vi "WM_CAP - AM Capture.vi"() -> ()   [LabVIEW 2022 SP3]
uses:
  System.Windows.Forms
  user32.dll
  avicap32.dll
panel:
  in  "Preview":bool
  in  "Export":bool
  in  "Capture":bool
  in  "Frame to BMP":bool
  in  "Copy Frame":bool
  in  "Capture FPS":dbl
  in  "Preview FPS":dbl
  in  "PictureBox":refnum<k24>(container)
  out "Info":string
  in  "Fit Window":bool
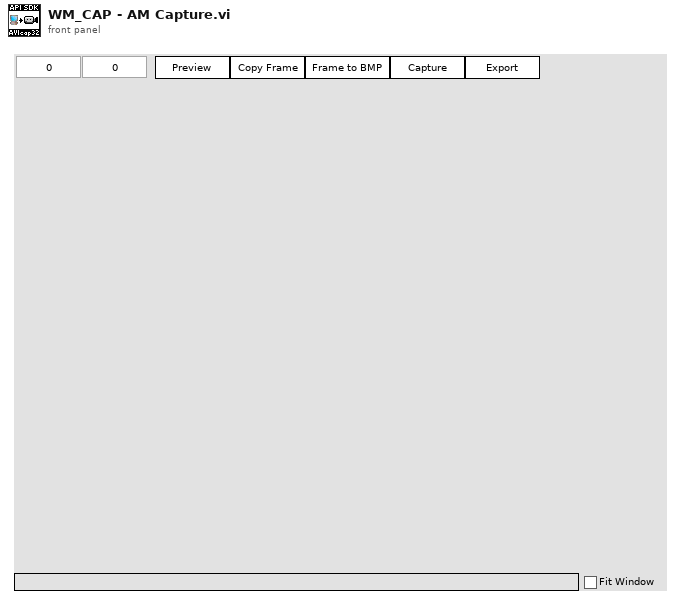
[diagram p1: front panel]
types:
  T1 = cluster{"biSize":i32, "biWidth":i32, "biHeight":i32, "biPlanes":i16, "biBitCount":i16, "biCompression":i32, "biSizeImage":i32, "biXPelsPerMeter":i32, "biYPelsPerMeter":i32, "biClrUsed":i32, "biClrImportant":i32, "Colors":u32[]}
  T2 = cluster{"uiImageWidth":u32, "uiImageHeight":u32, "fLiveWindow":u32, "fOverlayWindow":u32, "fScale":u32, "ptScroll":cluster{"x":i32, "y":i32}, "fUsingDefaultPalette":u32, "fAudioHardware":u32, "fCapFileExists":u32, "dwCurrentVideoFrame":u32, "dwCurrentVideoFramesDropped":u32, "dwCurrentWaveSamples":u32, "dwCurrentTimeElapsedMS":u32, "hPalCurrent":u32, "fCapturingNow":u32, "dwReturn":u32, "wNumVideoAllocated":u32, "wNumAudioAllocated":u32}
  T3 = cluster{"Timeout":i32, "Error":errorcluster, "hwnd":u32, "WM_CAP_START":u32, "CAPSTATUS":cluster{"uiImageWidth":u32, "uiImageHeight":u32, "fLiveWindow":u32, "fOverlayWindow":u32, "fScale":u32, "ptScroll":cluster{"x":i32, "y":i32}, "fUsingDefaultPalette":u32, "fAudioHardware":u32, "fCapFileExists":u32, "dwCurrentVideoFrame":u32, "dwCurrentVideoFramesDropped":u32, "dwCurrentWaveSamples":u32, "dwCurrentTimeElapsedMS":u32, "hPalCurrent":u32, "fCapturingNow":u32, "dwReturn":u32, "wNumVideoAllocated":u32, "wNumAudioAllocated":u32}, "BITMAPINFO":cluster{"biSize":i32, "biWidth":i32, "biHeight":i32, "biPlanes":i16, "biBitCount":i16, "biCompression":i32, "biSizeImage":i32, "biXPelsPerMeter":i32, "biYPelsPerMeter":i32, "biClrUsed":i32, "biClrImportant":i32, "Colors":u32[]}, "Preview FPS":dbl, "Capture FPS":dbl, "Camera":string}
  T4 = typedef "sizeaction.ctl" = enum32{"Minimized", "Maximized", "Resized"}
  T5 = typedef "LVRectTypeDef.ctl" = cluster{"Left":i16, "Top":i16, "Right":i16, "Bottom":i16}
  T6 = cluster{"wDeviceIndex":u32, "fHasOverlay":u32, "fHasDlgVideoSource":u32, "fHasDlgVideoFormat":u32, "fHasDlgVideoDisplay":u32, "fCaptureInitialized":u32, "fDriverSuppliesPalettes":u32, "hVideoIn":u32, "hVideoOut":u32, "hVideoExtIn":u32, "hVideoExtOut":u32}
  T7 = typedef "imagedata.ctl" = cluster{"image type":i32, "image depth":i32, "image":u8[], "mask":u8[], "colors":u32[], "Rectangle":cluster{"left":i16, "top":i16, "right":i16, "bottom":i16}}
  T8 = cluster{"dwRequestMicroSecPerFrame":u32, "fMakeUserHitOKToCapture":u32, "wPercentDropForError":u32, "fYield":u32, "dwIndexSize":u32, "wChunkGranularity":u32, "fUsingDOSMemory":u32, "wNumVideoRequested":u32, "fCaptureAudio":u32, "wNumAudioRequested":u32, "vKeyAbort":u32, "fAbortLeftMouse":u32, "fAbortRightMouse":u32, "fLimitEnabled":u32, "wTimeLimit":u32, "fMCIControl":u32, "fStepMCIDevice":u32, "dwMCIStartTime":u32, "dwMCIStopTime":u32, " fStepCaptureAt2x":u32, "wStepCaptureAverageFrames":u32, "dwAudioBufferSize":u32, "fDisableWriteCache":u32, "AVStreamMaster":u32}
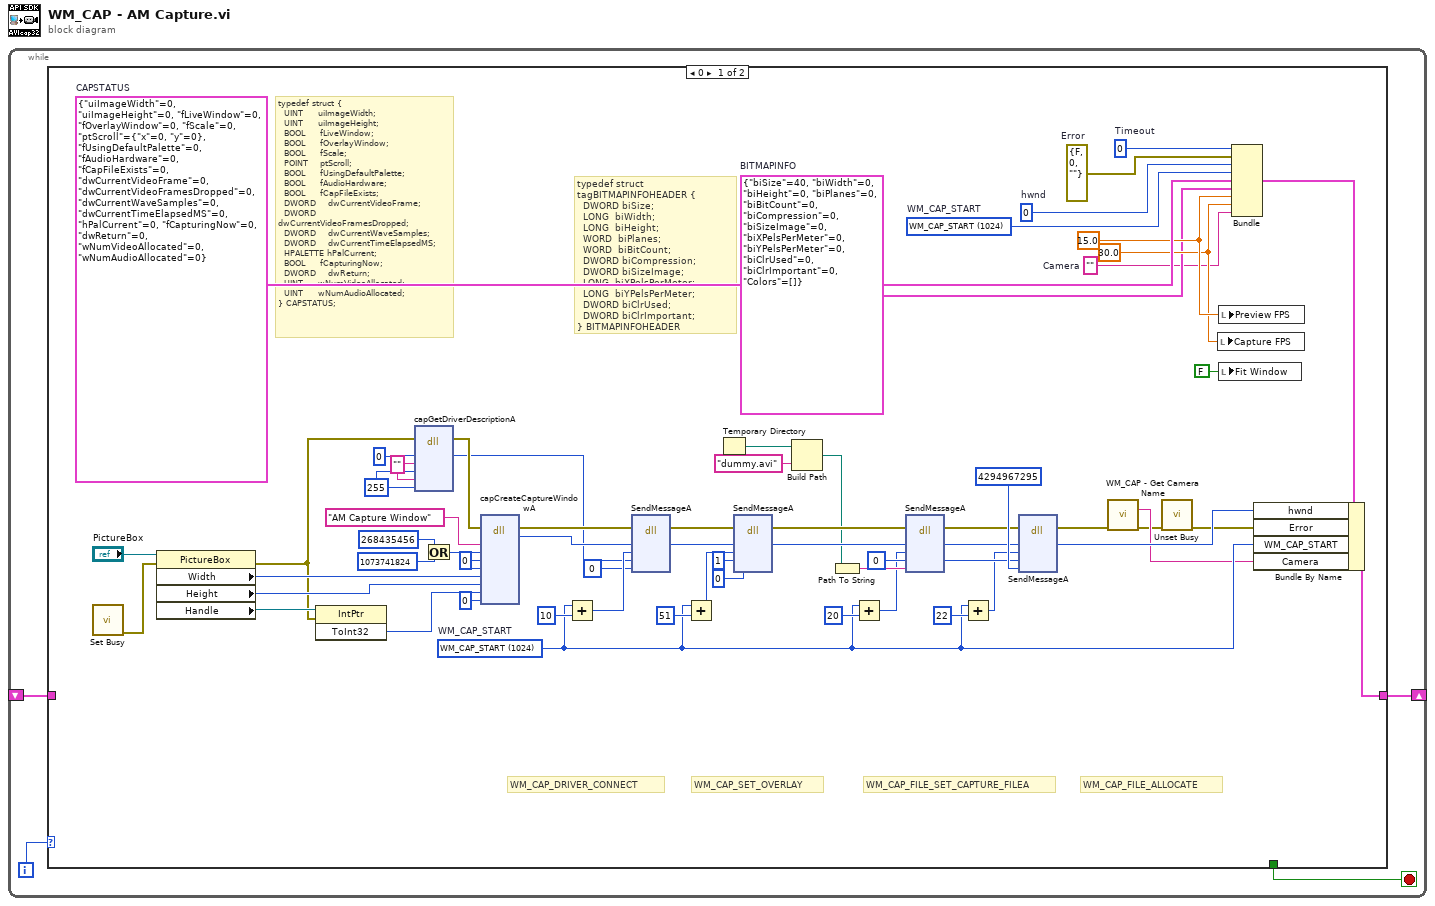
[diagram p0: block diagram]
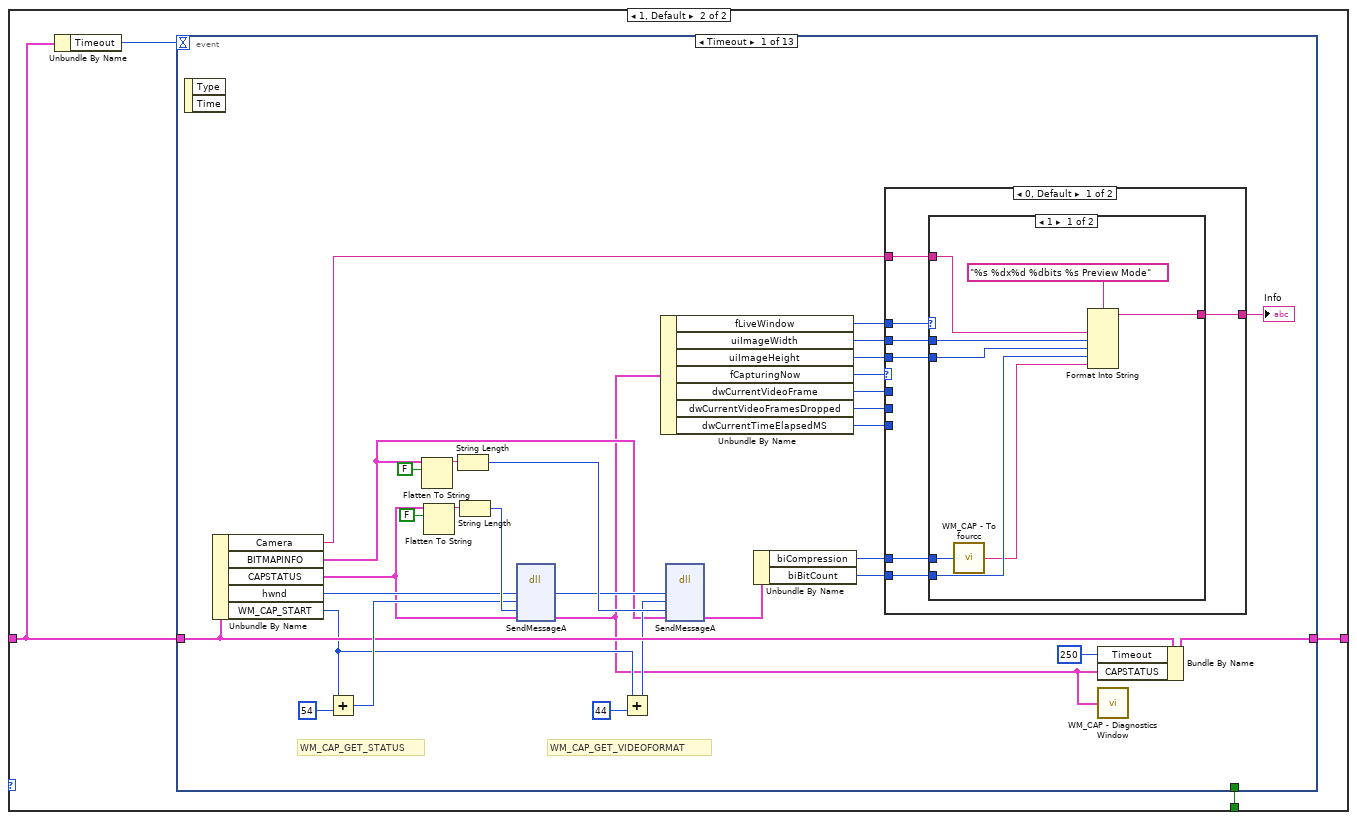
[diagram p2: hidden frame]
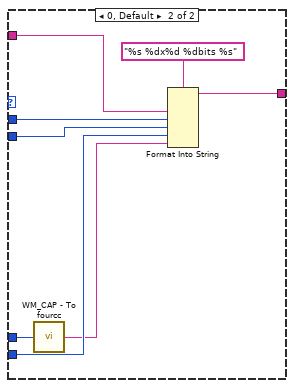
[diagram p3: hidden frame]
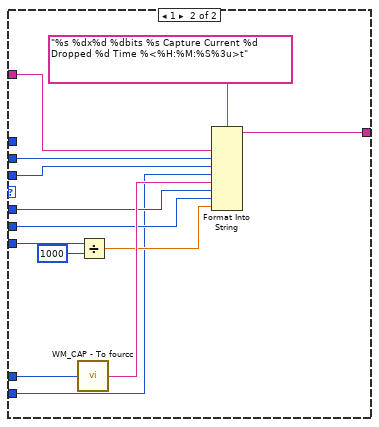
[diagram p4: hidden frame]
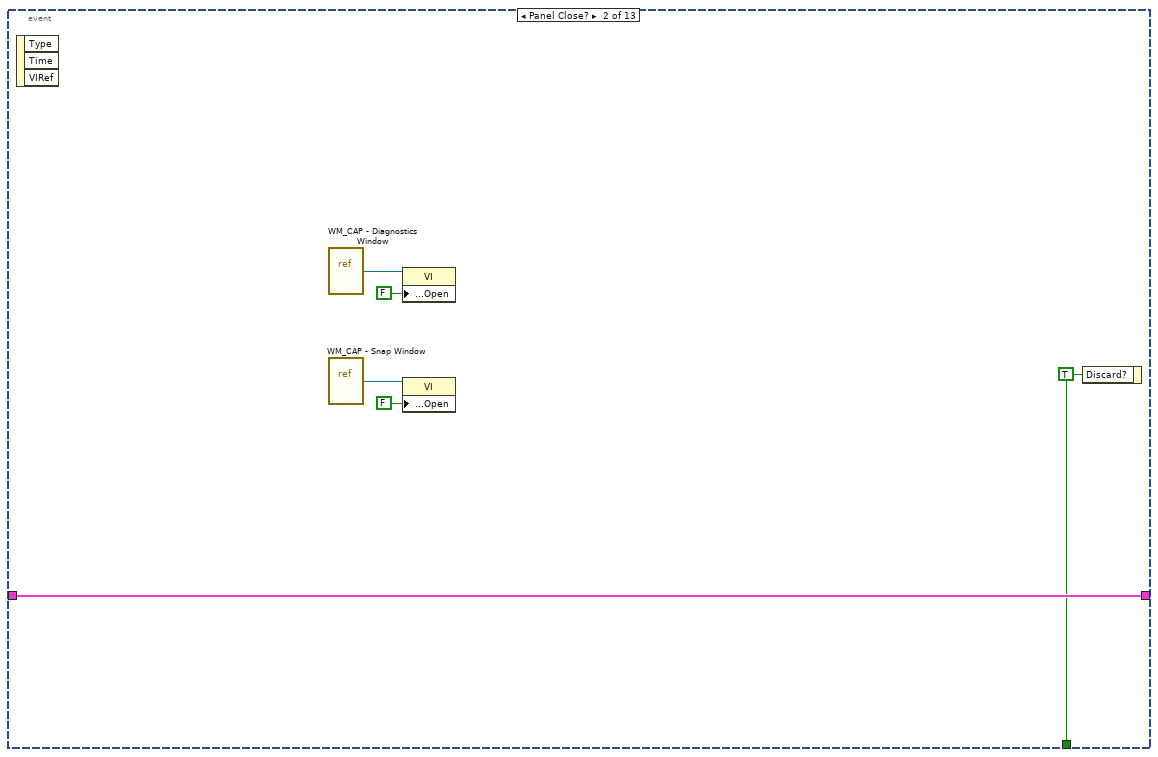
[diagram p5: hidden frame]
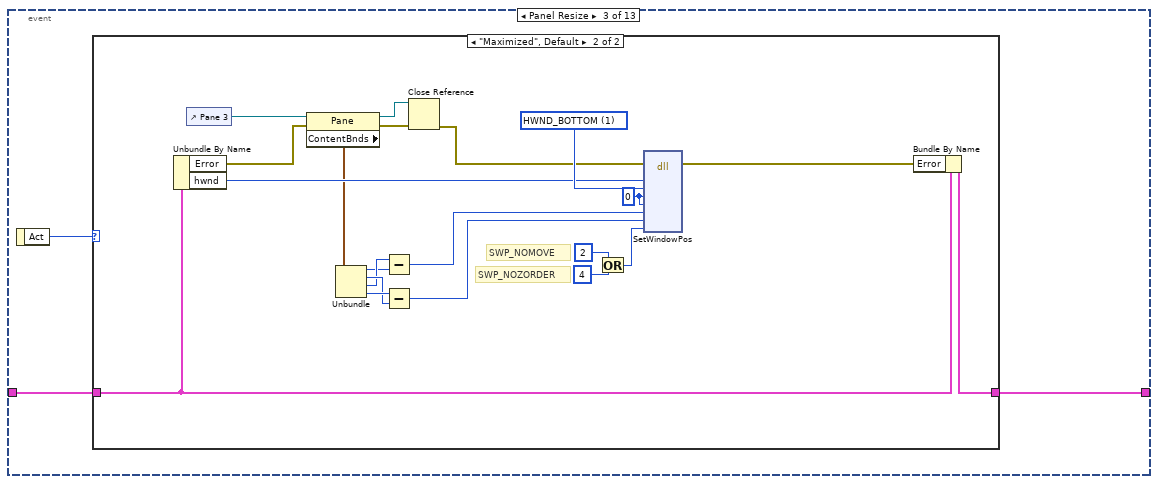
[diagram p6: hidden frame]
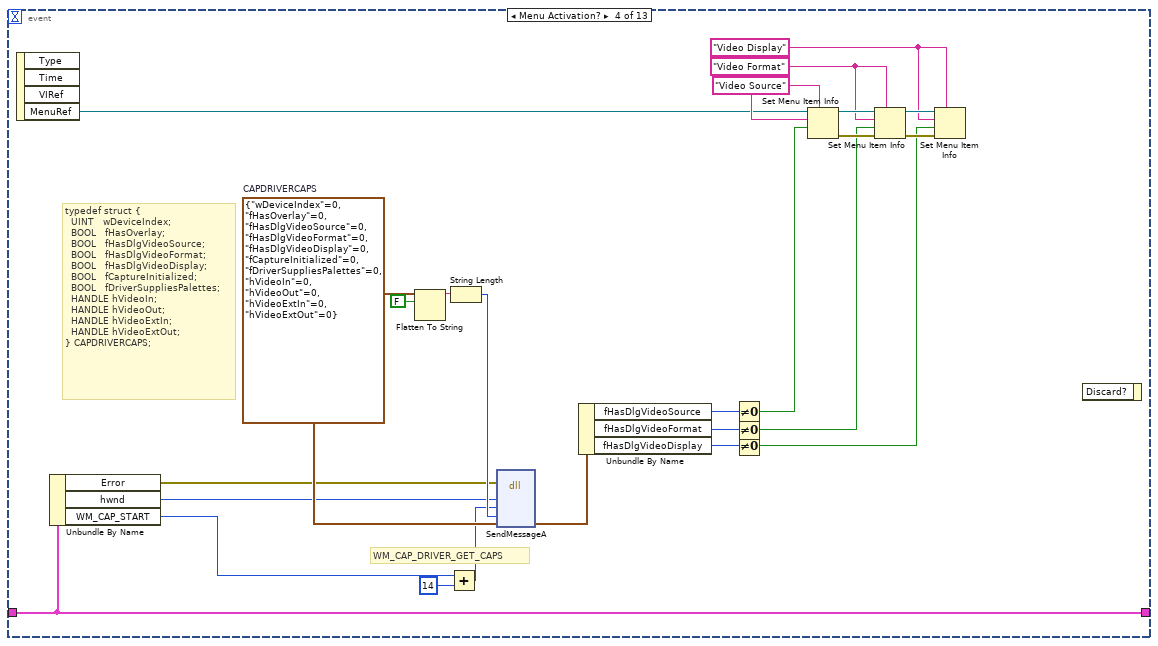
[diagram p8: hidden frame]
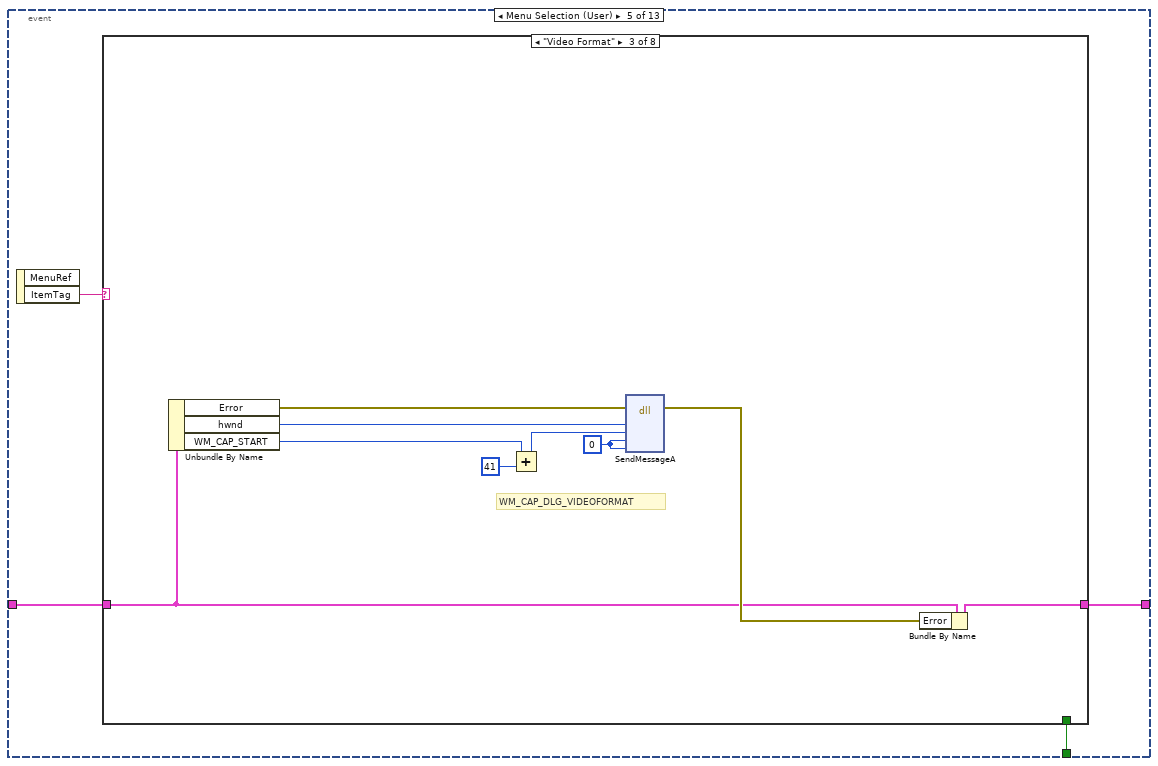
[diagram p9: hidden frame]
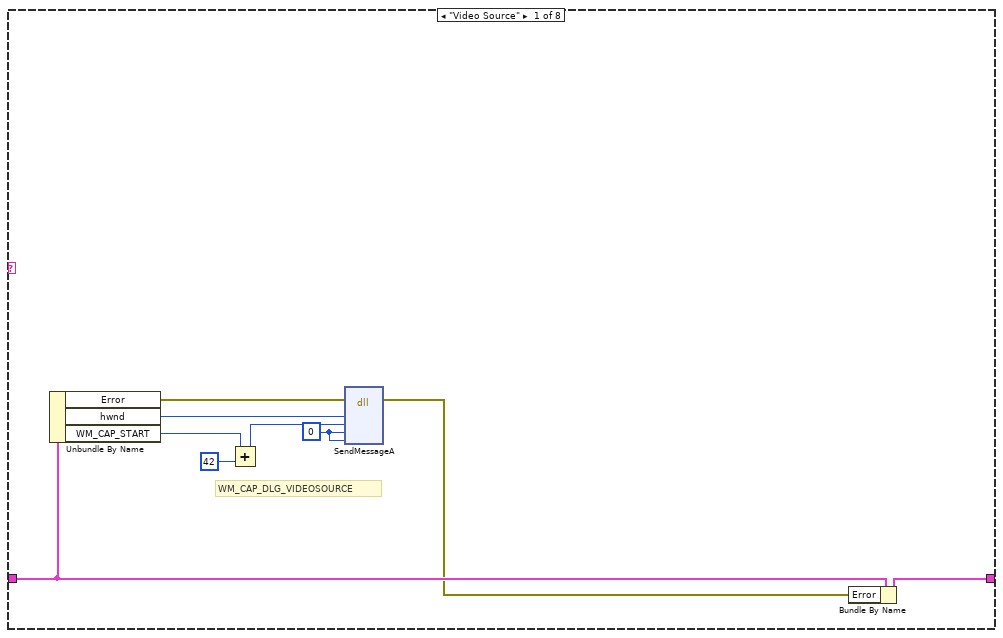
[diagram p10: hidden frame]
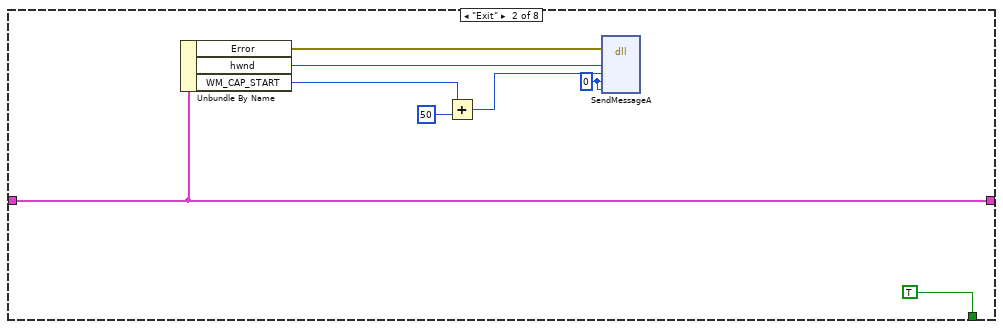
[diagram p11: hidden frame]
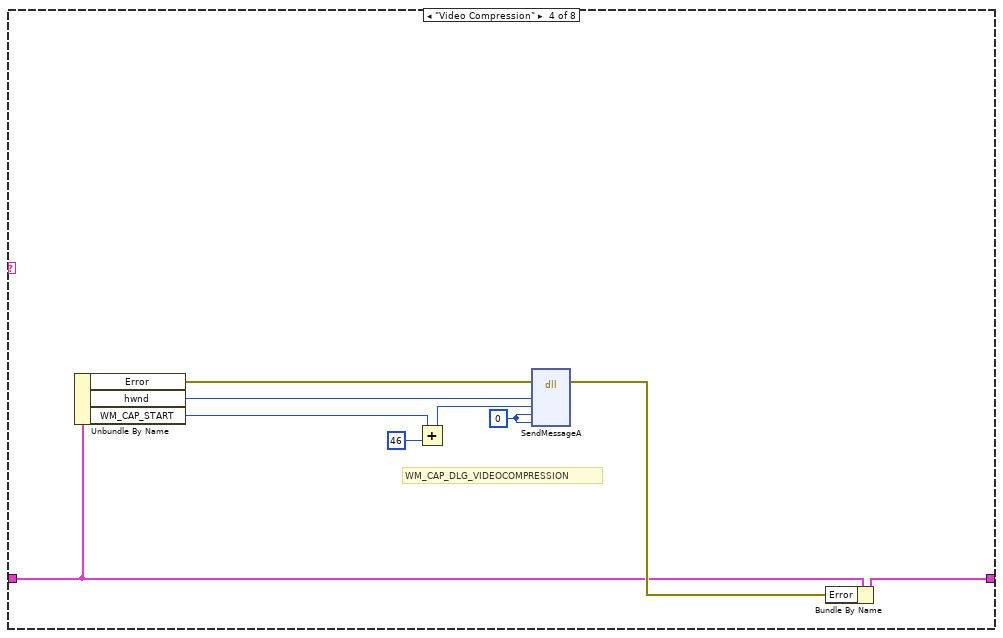
[diagram p12: hidden frame]
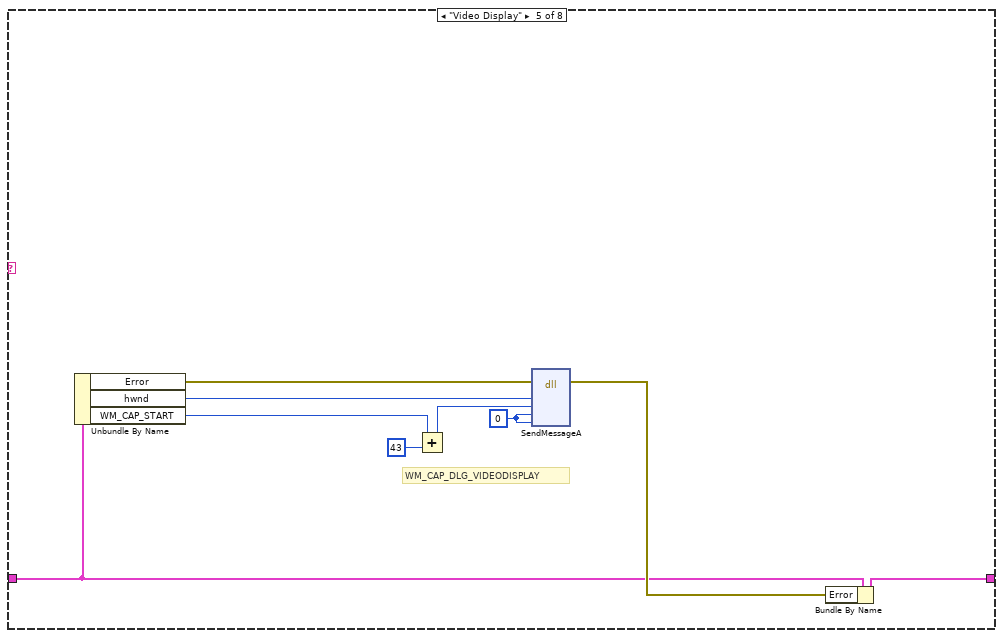
[diagram p13: hidden frame]
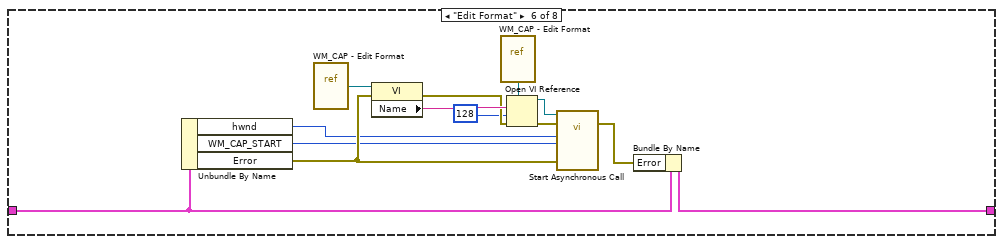
[diagram p14: hidden frame]
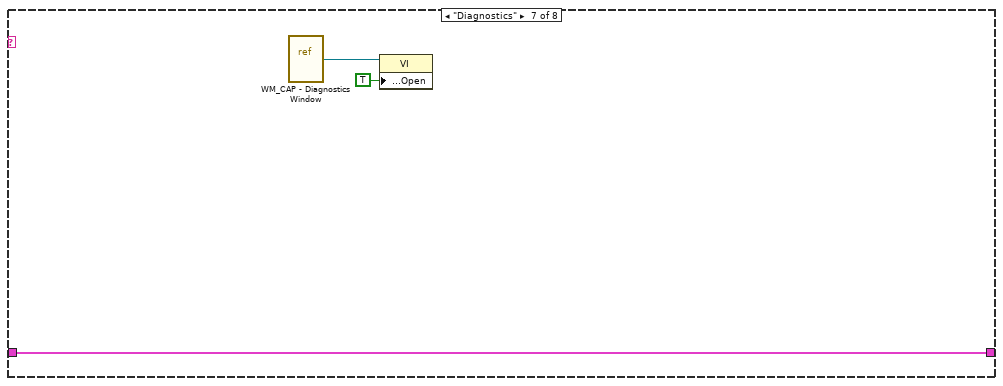
[diagram p15: hidden frame]
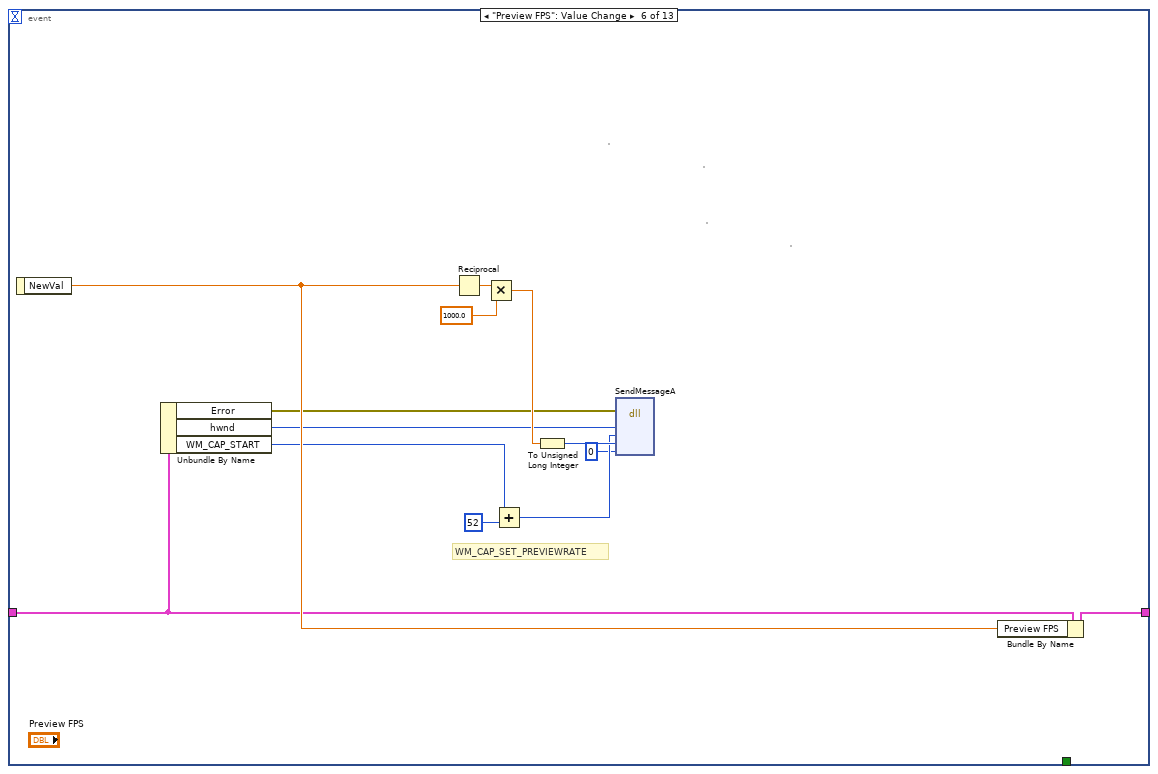
[diagram p17: hidden frame]
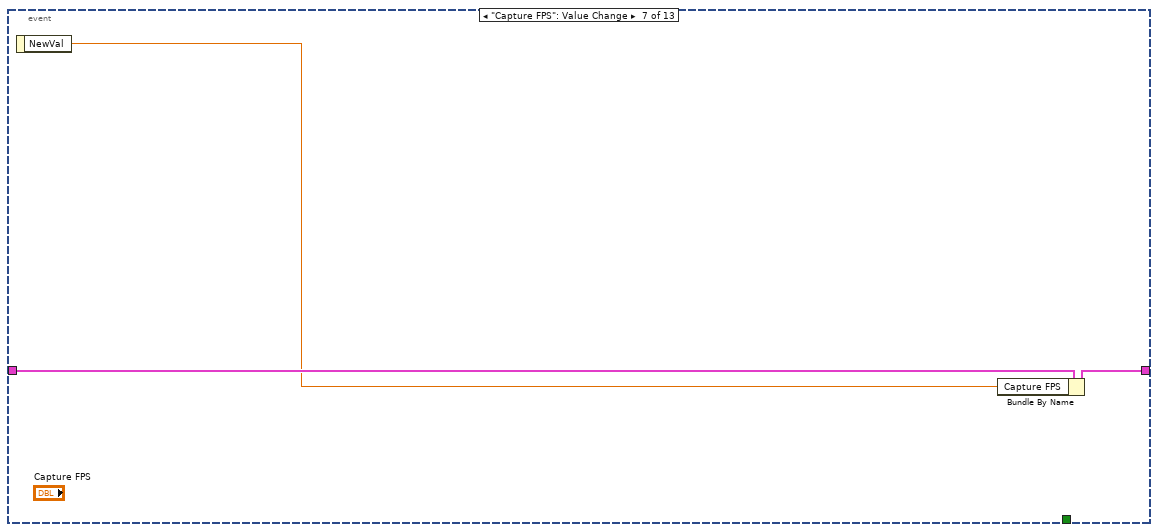
[diagram p18: hidden frame]
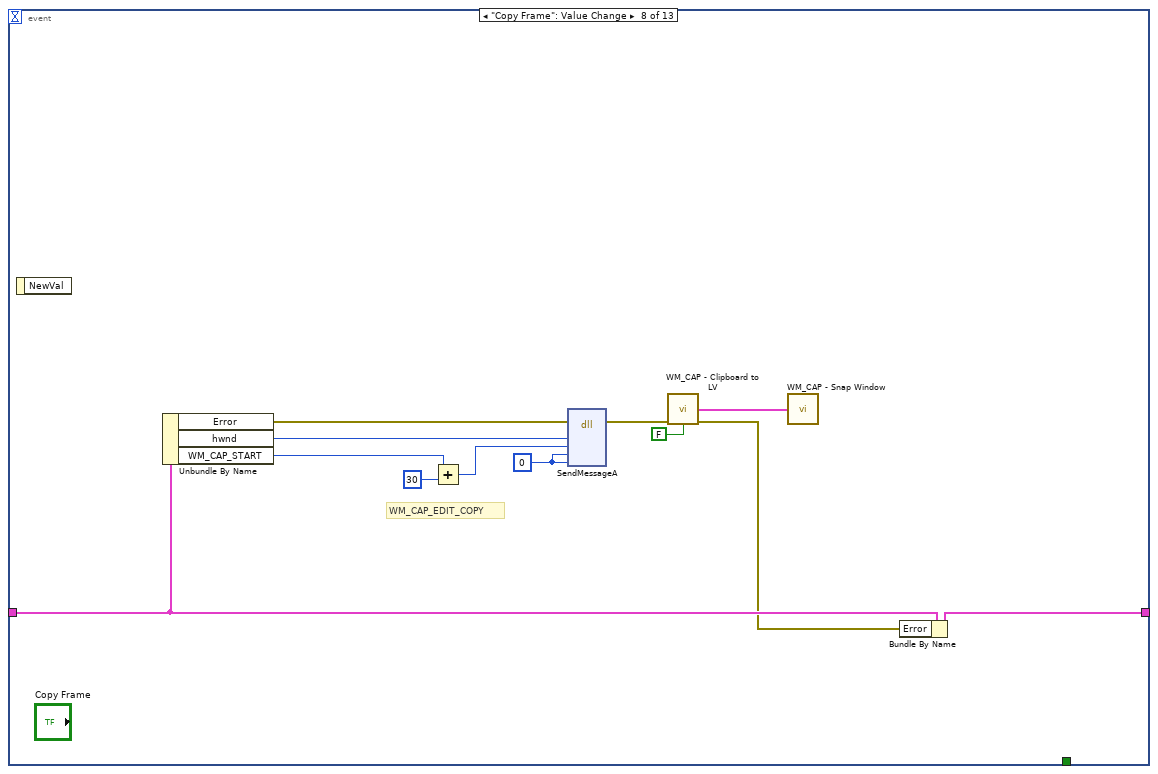
[diagram p19: hidden frame]
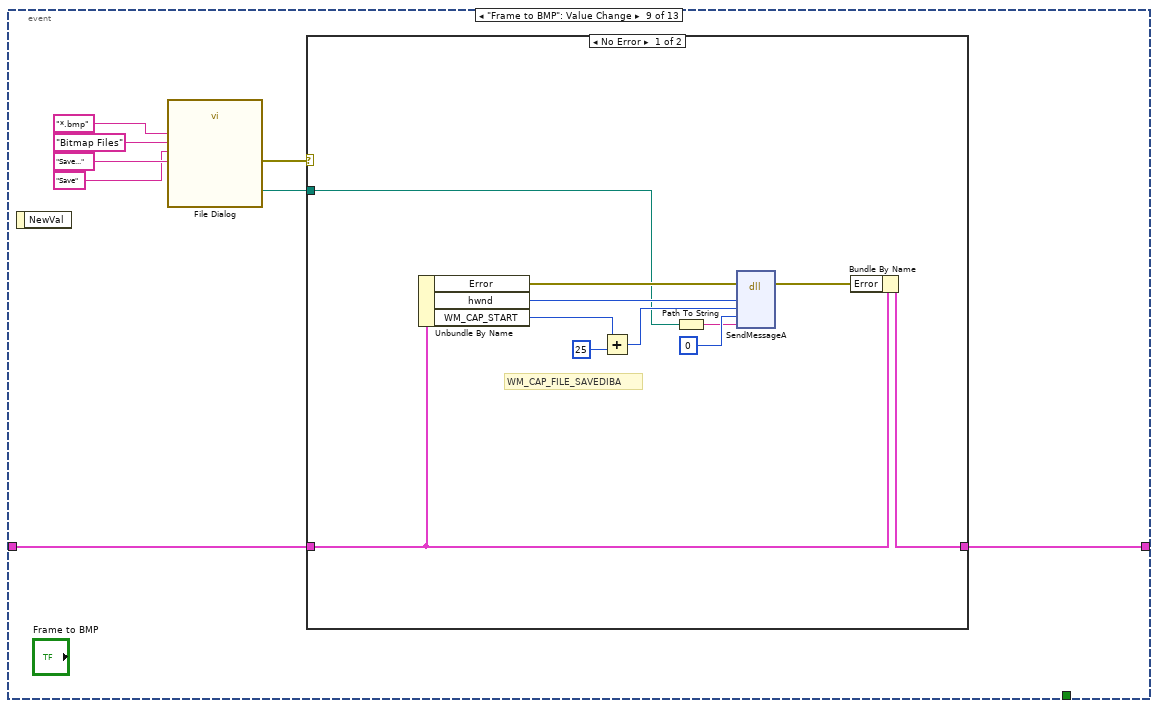
[diagram p20: hidden frame]
diagram:
  n1 = while {
    shift-right: [w3] -> _
    shift-left: _ -> [w2]
    i -> [w4]
    stop <- w1 stop-if-true
    n2 = case shown="0" w4 {
      tunnel: [w47 w70] -> w3
      tunnel: w2 -> [_ w69]
      tunnel: [_ w67] -> w1
      frame 0 {
        w8 = ""  # Camera
        w12 = T1 {"biSize"=40, "biWidth"=0, "biHeight"=0, "biPlanes"=0, "biBitCount"=0, "biCompression"=0, "biSizeImage"=0, "biXPelsPerMeter"=0, "biYPelsPerMeter"=0, "biClrUsed"=0, "biClrImportant"=0, "Colors"=[]}  # BITMAPINFO
        w17 = T2 {"uiImageWidth"=0, "uiImageHeight"=0, "fLiveWindow"=0, "fOverlayWindow"=0, "fScale"=0, "ptScroll"={"x"=0, "y"=0}, "fUsingDefaultPalette"=0, "fAudioHardware"=0, "fCapFileExists"=0, "dwCurrentVideoFrame"=0, "dwCurrentVideoFramesDropped"=0, "dwCurrentWaveSamples"=0, "dwCurrentTimeElapsedMS"=0, "hPalCurrent"=0, "fCapturingNow"=0, "dwReturn"=0, "wNumVideoAllocated"=0, "wNumAudioAllocated"=0}  # CAPSTATUS
        w14 = 30.0 ("Capture FPS")
        w15 = 15.0 ("Preview FPS")
        w22 = u32 1024 items=["WM_CAP_START"=1024]  # WM_CAP_START
        w23 = u32 1024 items=["WM_CAP_START"=1024]  # WM_CAP_START
        w48 = u32 0  # hwnd
        w55 = u32 0 ("x")
        w61 = 255 ("cbName")
        w62 = ""
        w65 = errorcluster {"status"=FALSE, "code"=0, "source"=""}  # Error
        w66 = 0  # Timeout
        # "typedef struct tagBITMAPINFOHEADER {\n  DWORD biSize;\n  LONG  biWidth;\n  LONG  biHeight;\n  WORD  biPlanes;\n  WORD  biBitCount;\n  DWORD biCompression;\n  DWORD biSizeImage;\n  LONG  biXPelsPerMeter;\n  LONG  biYPelsPerMeter;\n  DWORD biClrUsed;\n  DWORD biClrImportant;\n} BITMAPINFOHEADER"
        # "typedef struct {\n  UINT     uiImageWidth;\n  UINT     uiImageHeight;\n  BOOL     fLiveWindow;\n  BOOL     fOverlayWindow;\n  BOOL     fScale;\n  POINT    ptScroll;\n  BOOL     fUsingDefaultPalette;\n  BOOL     fAudioHardware;\n  BOOL     fCapFileExists;\n  DWORD    dwCurrentVideoFrame;\n  DWORD    dwCurrentVideoFramesDropped;\n  DWORD    dwCurrentWaveSamples;\n  DWORD    dwCurrentTimeElapsedMS;\n  HPALETTE hPalCurrent;\n  BOOL     fCapturingNow;\n  DWORD    dwReturn;\n  UINT     wNumVideoAllocated;\n  UINT     wNumAudioAllocated;\n} CAPSTATUS;"
        # "WM_CAP_FILE_ALLOCATE"
        # "WM_CAP_FILE_SET_CAPTURE_FILEA"
        # "WM_CAP_SET_OVERLAY"
        # "WM_CAP_DRIVER_CONNECT"
        n3 = call <vilib>:"Set Busy.vi"() -> ("error out"=w19:errorcluster)  [unwired: 10 in, 1 out]
        n4 = property class="PictureBox"(reference="PictureBox", error in=w19) -> (error out=w16:errorcluster, "Width"=w59:i32, "Height"=w60:i32, "Handle"=w57:refnum<k24>)  [unwired: 1 out]
        n5 = invoke class="IntPtr" method="ToInt32"(reference=w57, error in=w16) -> ("ToInt32"=w58:i32)  [unwired: 1 in, 2 out]
        n6 = dll-call lib="avicap32.dll" fn="capGetDriverDescriptionA"(error in=w16, "wDriverIndex"=0, "lpszName"=w62, "cbName"=w61, "lpszVer"=w62, "cbVer"=w61) -> (error out=w49:errorcluster, "wDriverIndex"=w20:i32)  [unwired: 7 in, 1 out]
        n7 = Or(x=u32 268435456, y=u32 1073741824) -> (x .or. y?=w54:u32)
        n8 = dll-call lib="avicap32.dll" fn="capCreateCaptureWindowA"(error in=w49, "lpszWindowName"="AM Capture Window", "dwStyle"=w54, "x"=w55, "y"=w55, "nWidth"=w59, "nHeight"=w60, "hwnd"=w58, "nID"=u32 0) -> (error out=w46:errorcluster, "return type"=w44:u32)  [unwired: 10 in, 1 out]
        n9 = Add(x=w23, y=u32 10) -> (x+y=w43:u32)
        n10 = dll-call lib="user32.dll" fn="SendMessageA"(error in=w46, "hwnd"=w44, "msg"=w43, "wParam"=w20, "lparam"=u32 0 ("msg")) -> (error out=w39:errorcluster, "hwnd"=w37:u32)  [unwired: 6 in, 1 out]
        n11 = Add(x=w23, y=u32 51) -> (x+y=w36:u32)
        n12 = Temporary Directory() -> (w11:path)
        n13 = dll-call lib="user32.dll" fn="SendMessageA"(error in=w39, "hwnd"=w37, "msg"=w36, "wParam"=u32 1, "lparam"=u32 0) -> (error out=w25:errorcluster, "hwnd"=w21:u32)  [unwired: 6 in, 1 out]
        n14 = Build Path(base path=w11, name or relative path="dummy.avi") -> (appended path=w9:path)
        n15 = Path To String(path=w9) -> (string=w29:string)
        n16 = Add(x=w23, y=u32 20) -> (x+y=w27:u32)
        n17 = dll-call lib="user32.dll" fn="SendMessageA"(error in=w25, "hwnd"=w21, "msg"=w27, "wParam"=u32 0 ("msg"), "lparam"=w29) -> (error out=w30:errorcluster, "hwnd"=w31:u32, "wParam"=w34:u32)  [unwired: 5 in, 1 out]
        n18 = Add(x=w23, y=u32 22) -> (x+y=w33:u32)
        n19 = dll-call lib="user32.dll" fn="SendMessageA"(error in=w30, "hwnd"=w31, "msg"=w33, "wParam"=w34, "lparam"=u32 4294967295) -> (error out=w6:errorcluster, "hwnd"=w24:u32)  [unwired: 6 in, 1 out]
        n20 = call "WM_CAP - Get Camera Name.vi"("error in (no error)"=w6) -> ("FriendlyName"=w7:string, "error out"=w5:errorcluster)  [unwired: 12 in, 1 out]
        n21 = call <vilib>:"Unset Busy.vi"("error in (no error)"=w5) -> ("error out"=w18:errorcluster)  [unwired: 10 in]
        n22 = local write "Capture FPS"(w14) -> ()
        n23 = local write "Preview FPS"(w15) -> ()
        n24 = local write "Fit Window"(FALSE ("Fit Window")) -> ()
        n25 = Bundle("Timeout"=w66, "Error"=w65, "hwnd"=w48, "WM_CAP_START"=w22, "CAPSTATUS"=w17, "BITMAPINFO"=w12, "Preview FPS"=w15, "Capture FPS"=w14, "Camera"=w8) -> (w64:T3)  [unwired: 1 in]
        n26 = Bundle By Name(cluster=w64, "hwnd"=w24, "Error"=w18, "WM_CAP_START"=w23, "Camera"=w7) -> (w47:T3)
      }
      frame 1, Default {
        n27 = Unbundle By Name(w69) -> ("Timeout"=w68:i32)
        n28 = event shown="[0] Timeout" {
          selector: _ -> [_ _ _ _ _ _ _ _ _ _ _ _ _]
          dyn-events: _ -> [_ _ _ _ _ _ _ _ _ _ _ _ _]
          timeout: w68 -> [_ _ _ _ _ _ _ _ _ _ _ _ _]
          tunnel: [w101 w143 w145 w184 w196 w271 w273 w279 w293 w308 w361 w381 w415] -> w70
          tunnel: w69 -> [w94 w143 w146 w184 w195 w262 w274 w283 w294 w309 w362 w382 w415]
          tunnel: [_ w142 _ _ w194 _ _ _ _ _ _ _ _] -> w67
          event Timeout {
            # "WM_CAP_GET_VIDEOFORMAT"
            # "WM_CAP_GET_STATUS"
            n29 = event-data() -> ()  [unwired: 1 in, 2 out]
            n30 = Unbundle By Name(w94) -> ("Camera"=w71:string, "BITMAPINFO"=w81:T1, "CAPSTATUS"=w92:T2, "hwnd"=w93:u32, "WM_CAP_START"=w82:u32)
            n31 = Add(x=w82, y=u32 54) -> (x+y=w96:u32)
            n32 = Flatten To String(anything=w81, prepend array or string size? (T)=FALSE) -> (data string=w87:string)  [unwired: 2 in, 2 out]
            n33 = Flatten To String(anything=w92, prepend array or string size? (T)=FALSE) -> (data string=w97:string)  [unwired: 2 in, 2 out]
            n34 = String Length(string=w87) -> (length=w85:i32)
            n35 = String Length(string=w97) -> (length=w99:i32)
            n36 = dll-call lib="user32.dll" fn="SendMessageA"("hwnd"=w93, "msg"=w96, "wParam"=w99, w92) -> ("hwnd"=w83:u32, w80:T2)  [unwired: 6 in, 2 out]
            n37 = Add(x=w82, y=u16 44) -> (x+y=w84:u32)
            n38 = Unbundle By Name(w80) -> ("fLiveWindow"=w75:u32, "uiImageWidth"=w90:u32, "uiImageHeight"=w89:u32, "fCapturingNow"=w91:u32, "dwCurrentVideoFrame"=w74:u32, "dwCurrentVideoFramesDropped"=w73:u32, "dwCurrentTimeElapsedMS"=w72:u32)
            n39 = dll-call lib="user32.dll" fn="SendMessageA"("hwnd"=w83, "msg"=w84, "wParam"=w85, "lparam"=w81) -> ("lparam"=w79:T1)  [unwired: 7 in, 2 out]
            n40 = Unbundle By Name(w79) -> ("biCompression"=w78:i32, "biBitCount"=w77:i16)
            n41 = case shown="0, Default" w91 {
              tunnel: w90 -> [w108 w131]
              tunnel: w89 -> [w107 w130]
              tunnel: w78 -> [w105 w137]
              tunnel: w77 -> [w106 w125]
              tunnel: [w104 w136] -> w76
              tunnel: w75 -> [w103 _]
              tunnel: w74 -> [_ w126]
              tunnel: w73 -> [_ w127]
              tunnel: w72 -> [_ w134]
              tunnel: w71 -> [w102 w132]
              frame 0, Default {
                n42 = case shown="1" w103 {
                  tunnel: w108 -> [w112 w120]
                  tunnel: w107 -> [w111 w119]
                  tunnel: w106 -> [w110 w118]
                  tunnel: w105 -> [w115 w123]
                  tunnel: [w114 w122] -> w104
                  tunnel: w102 -> [w113 w121]
                  frame 1 {
                    n43 = call "WM_CAP - To fourcc.vi"("biCompression"=w115) -> ("FOURCC"=w109:string)  [unwired: 14 in]
                    n44 = Format Into String(format string="%s %dx%d %dbits %s Preview Mode", w113, w112, w111, w110, w109) -> (resulting string=w114:string)  [unwired: 2 in, 1 out]
                  }
                  frame 0, Default {
                    n45 = call "WM_CAP - To fourcc.vi"("biCompression"=w123) -> ("FOURCC"=w117:string)  [unwired: 14 in]
                    n46 = Format Into String(format string="%s %dx%d %dbits %s", w121, w120, w119, w118, w117) -> (resulting string=w122:string)  [unwired: 2 in, 1 out]
                  }
                }
              }
              frame 1 {
                n47 = call "WM_CAP - To fourcc.vi"("biCompression"=w137) -> ("FOURCC"=w129:string)  [unwired: 14 in]
                n48 = Divide(x=w134, y=u32 1000) -> (x/y=w128:dbl)
                n49 = Format Into String(format string="%s %dx%d %dbits %s Capture Current %d Dropped %d Time %<%H:%M:%S%3u>t", w132, w131, w130, w125, w129, w126, w127, w128) -> (resulting string=w136:string)  [unwired: 2 in, 1 out]
              }
            }
            "Info" <- w76
            n50 = Bundle By Name(cluster=w94, "Timeout"=250, "CAPSTATUS"=w80) -> (w101:T3)
            n51 = call "WM_CAP - Diagnostics Window.vi"("CAPSTATUS In"=w80) -> ()  [unwired: 15 in]
          }
          event Panel Close? {
            w142 = TRUE ("Discard?")
            n52 = event-data() -> ()  [unwired: 1 in, 3 out]
            n53 = vi-ref "WM_CAP - Diagnostics Window.vi"() -> (w141:refnum<vi>)
            n54 = vi-ref "WM_CAP - Snap Window.vi"() -> (w138:refnum<vi>)
            n55 = property class="VI"(reference=w141, "Front Panel.Open"=FALSE ("Front Panel Window:Open")) -> ()  [unwired: 1 in, 2 out]
            n56 = property class="VI"(reference=w138, "Front Panel.Open"=FALSE ("Front Panel Window:Open")) -> ()  [unwired: 1 in, 2 out]
            n57 = event-data("Discard?"=w142) -> ()  [unwired: 1 in, 1 out]
          }
          event Panel Resize {
            n58 = event-data() -> ("Act"=w144:T4)  [unwired: 1 in]
            n59 = case shown="\"Maximized\", Default" w144 {
              tunnel: w146 -> [w147 w164]
              tunnel: [w147 w162] -> w145
              frame "Minimized" {
              }
              frame "Maximized", Default {
                w151 = u32 0 ("x")
                w167 = 1 items=["HWND_BOTTOM"=1, "HWND_NOTOPMOST"=-2, "HWND_TOP"=0, "HWND_TOPMOST"=-1] ("hwndInsertAfter")
                # "SWP_NOMOVE"
                # "SWP_NOZORDER"
                n60 = Unbundle By Name(w164) -> ("Error"=w155:errorcluster, "hwnd"=w163:u32)
                n61 = control-ref of="Pane 3"() -> (w148:refnum<vi>)
                n62 = property class="Pane"(reference=w148, error in=w155) -> (reference out=w154:refnum<vi>, error out=w153:errorcluster, "ContentBnds"=w160:T5)
                n63 = Unbundle(w160) -> ("Left"=w156:i16, "Top"=w158:i16, "Right"=w157:i16, "Bottom"=w159:i16)
                n64 = Subtract(x=w157, y=w156) -> (x-y=w150:i16)
                n65 = Subtract(x=w159, y=w158) -> (x-y=w149:i16)
                n66 = Close Reference(reference=w154, error in (no error)=w153) -> (error out=w152:errorcluster)
                n67 = Or(x=u32 2, y=u32 4) -> (x .or. y?=w168:u32)
                n68 = dll-call lib="user32.dll" fn="SetWindowPos"(error in=w152, "hwnd"=w163, "hwndInsertAfter"=w167, "x"=w151, "y"=w151, "cx"=w150, "cy"=w149, "uFlags"=w168) -> (error out=w161:errorcluster)  [unwired: 10 in, 1 out]
                n69 = Bundle By Name(cluster=w164, "Error"=w161) -> (w162:T3)
              }
            }
          }
          event Menu Activation? {
            w176 = "Video Display" ("item tag")
            w177 = "Video Format" ("item tag")
            w178 = "Video Source" ("item tag")
            w192 = T6 {"wDeviceIndex"=0, "fHasOverlay"=0, "fHasDlgVideoSource"=0, "fHasDlgVideoFormat"=0, "fHasDlgVideoDisplay"=0, "fCaptureInitialized"=0, "fDriverSuppliesPalettes"=0, "hVideoIn"=0, "hVideoOut"=0, "hVideoExtIn"=0, "hVideoExtOut"=0}  # CAPDRIVERCAPS
            # "WM_CAP_DRIVER_GET_CAPS"
            # "typedef struct {\n  UINT   wDeviceIndex;\n  BOOL   fHasOverlay;\n  BOOL   fHasDlgVideoSource;\n  BOOL   fHasDlgVideoFormat;\n  BOOL   fHasDlgVideoDisplay;\n  BOOL   fCaptureInitialized;\n  BOOL   fDriverSuppliesPalettes;\n  HANDLE hVideoIn;\n  HANDLE hVideoOut;\n  HANDLE hVideoExtIn;\n  HANDLE hVideoExtOut;\n} CAPDRIVERCAPS;"
            n70 = event-data() -> ("MenuRef"=w169:refnum<k9>)  [unwired: 1 in, 3 out]
            n71 = Unbundle By Name(w184) -> ("Error"=w187:errorcluster, "hwnd"=w186:u32, "WM_CAP_START"=w185:u32)
            n72 = Flatten To String(anything=w192, prepend array or string size? (T)=FALSE) -> (data string=w190:string)  [unwired: 2 in, 2 out]
            n73 = Add(x=w185, y=u32 14) -> (x+y=w189:u32)
            n74 = String Length(string=w190) -> (length=w193:i32)
            n75 = dll-call lib="user32.dll" fn="SendMessageA"(error in=w187, "hwnd"=w186, "msg"=w189, "wParam"=w193, "lparam"=w192) -> ("lparam"=w181:T6)  [unwired: 6 in, 2 out]
            n76 = Unbundle By Name(w181) -> ("fHasDlgVideoSource"=w175:u32, "fHasDlgVideoFormat"=w174:u32, "fHasDlgVideoDisplay"=w173:u32)
            n77 = Not Equal To 0?(x=w175) -> (x != 0?=w172:bool)
            n78 = Not Equal To 0?(x=w174) -> (x != 0?=w171:bool)
            n79 = Not Equal To 0?(x=w173) -> (x != 0?=w170:bool)
            n80 = Set Menu Item Info(7:w178, 9:w172, 10:w178, 11:w169) -> (0:w183:errorcluster, 3:w180:refnum<k9>)  [unwired: 3 in]
            n81 = Set Menu Item Info(7:w177, 8:w183, 9:w171, 10:w177, 11:w180) -> (0:w182:errorcluster, 3:w179:refnum<k9>)  [unwired: 2 in]
            n82 = Set Menu Item Info(7:w176, 8:w182, 9:w170, 10:w176, 11:w179) -> ()  [unwired: 2 in, 2 out]
            n83 = event-data() -> ()  [unwired: 2 in, 1 out]
          }
          event Menu Selection (User) {
            n84 = event-data() -> ("ItemTag"=w197:string)  [unwired: 1 in, 1 out]
            n85 = case shown="\"Video Format\"" w197 {
              tunnel: [w201 w211 w220 w229 w238 w253 w257 w258] -> w196
              tunnel: w195 -> [w203 w211 w218 w227 w236 w254 w257 w258]
              tunnel: [_ TRUE _ _ _ _ _ _] -> w194
              frame "Video Source" {
                w206 = u32 0 ("msg")
                # "WM_CAP_DLG_VIDEOSOURCE"
                n86 = Unbundle By Name(w203) -> ("Error"=w199:errorcluster, "hwnd"=w198:u32, "WM_CAP_START"=w202:u32)
                n87 = Add(x=w202, y=u32 42) -> (x+y=w205:u32)
                n88 = dll-call lib="user32.dll" fn="SendMessageA"(error in=w199, "hwnd"=w198, "msg"=w205, "wParam"=w206, "lparam"=w206) -> (error out=w200:errorcluster)  [unwired: 7 in, 1 out]
                n89 = Bundle By Name(cluster=w203, "Error"=w200) -> (w201:T3)
              }
              frame "Exit" {
                w207 = u32 0 ("wParam")
                n90 = Unbundle By Name(w211) -> ("Error"=w210:errorcluster, "hwnd"=w209:u32, "WM_CAP_START"=w208:u32)
                n91 = Add(x=w208, y=u32 50) -> (x+y=w213:u32)
                n92 = dll-call lib="user32.dll" fn="SendMessageA"(error in=w210, "hwnd"=w209, "msg"=w213, "wParam"=w207, "lparam"=w207) -> ()  [unwired: 7 in, 2 out]
              }
              frame "Video Format" {
                w223 = u32 0 ("msg")
                # "WM_CAP_DLG_VIDEOFORMAT"
                n93 = Unbundle By Name(w218) -> ("Error"=w215:errorcluster, "hwnd"=w216:u32, "WM_CAP_START"=w217:u32)
                n94 = Add(x=w217, y=u32 41) -> (x+y=w222:u32)
                n95 = dll-call lib="user32.dll" fn="SendMessageA"(error in=w215, "hwnd"=w216, "msg"=w222, "wParam"=w223, "lparam"=w223) -> (error out=w219:errorcluster)  [unwired: 7 in, 1 out]
                n96 = Bundle By Name(cluster=w218, "Error"=w219) -> (w220:T3)
              }
              frame "Video Compression" {
                w232 = u32 0 ("msg")
                # "WM_CAP_DLG_VIDEOCOMPRESSION"
                n97 = Unbundle By Name(w227) -> ("Error"=w224:errorcluster, "hwnd"=w225:u32, "WM_CAP_START"=w226:u32)
                n98 = Add(x=w226, y=u32 46) -> (x+y=w231:u32)
                n99 = dll-call lib="user32.dll" fn="SendMessageA"(error in=w224, "hwnd"=w225, "msg"=w231, "wParam"=w232, "lparam"=w232) -> (error out=w228:errorcluster)  [unwired: 7 in, 1 out]
                n100 = Bundle By Name(cluster=w227, "Error"=w228) -> (w229:T3)
              }
              frame "Video Display" {
                w241 = u32 0 ("msg")
                # "WM_CAP_DLG_VIDEODISPLAY"
                n101 = Unbundle By Name(w236) -> ("Error"=w233:errorcluster, "hwnd"=w234:u32, "WM_CAP_START"=w235:u32)
                n102 = Add(x=w235, y=u32 43) -> (x+y=w240:u32)
                n103 = dll-call lib="user32.dll" fn="SendMessageA"(error in=w233, "hwnd"=w234, "msg"=w240, "wParam"=w241, "lparam"=w241) -> (error out=w237:errorcluster)  [unwired: 7 in, 1 out]
                n104 = Bundle By Name(cluster=w236, "Error"=w237) -> (w238:T3)
              }
              frame "Edit Format" {
                n105 = Unbundle By Name(w254) -> ("hwnd"=w243:u32, "WM_CAP_START"=w242:u32, "Error"=w244:errorcluster)
                n106 = vi-ref "WM_CAP - Edit Format.vi"() -> (w252:refnum<vi>)
                n107 = property class="VI"(reference=w252, error in=w244) -> (error out=w250:errorcluster, "Name"=w251:string)  [unwired: 1 out]
                n108 = vi-ref "WM_CAP - Edit Format.vi"() -> (w249:refnum<vi>)
                n109 = Open VI Reference(type specifier VI Refnum (for type only)=w249, vi path=w251, options=128, error in (no error)=w250) -> (vi reference=w246:refnum<vi>, error out=w247:errorcluster)  [unwired: 2 in]
                n110 = call-by-ref "Start Asynchronous Call"(reference=w246, error in=w247, "hwnd"=w243, "WM_CAP_START"=w242, "Error"=w244) -> (error out=w245:errorcluster)  [unwired: 12 in, 2 out]
                n111 = Bundle By Name(cluster=w254, "Error"=w245) -> (w253:T3)
              }
              frame "Diagnostics" {
                n112 = vi-ref "WM_CAP - Diagnostics Window.vi"() -> (w256:refnum<vi>)
                n113 = property class="VI"(reference=w256, "Front Panel.Open"=TRUE ("Front Panel Window:Open")) -> ()  [unwired: 1 in, 2 out]
              }
              frame "Error", Default {
              }
            }
          }
          event "Preview FPS": Value Change {
            # "WM_CAP_SET_PREVIEWRATE"
            n114 = event-data() -> ("NewVal"=w263:dbl)  [unwired: 1 in]
            n115 = Unbundle By Name(w262) -> ("Error"=w261:errorcluster, "hwnd"=w260:u32, "WM_CAP_START"=w259:u32)
            n116 = Reciprocal(x=w263) -> (1/x=w267:dbl)
            n117 = Multiply(x=w267, y=1000.0) -> (x*y=w269:dbl)
            n118 = Add(x=w259, y=u32 52) -> (x+y=w266:u32)
            n119 = To Unsigned Long Integer(number=w269) -> (unsigned 32bit integer=w270:u32)
            n120 = dll-call lib="user32.dll" fn="SendMessageA"(error in=w261, "hwnd"=w260, "msg"=w266, "wParam"=w270, "lparam"=u32 0) -> ()  [unwired: 7 in, 2 out]
            n121 = Bundle By Name(cluster=w262, "Preview FPS"=w263) -> (w271:T3)
          }
          event "Capture FPS": Value Change {
            n122 = event-data() -> ("NewVal"=w272:dbl)  [unwired: 1 in]
            n123 = Bundle By Name(cluster=w274, "Capture FPS"=w272) -> (w273:T3)
          }
          event "Copy Frame": Value Change {
            w286 = u32 0 ("msg")
            # "WM_CAP_EDIT_COPY"
            n124 = event-data() -> ()  [unwired: 1 in, 1 out]
            n125 = Unbundle By Name(w283) -> ("Error"=w282:errorcluster, "hwnd"=w281:u32, "WM_CAP_START"=w280:u32)
            n126 = Add(x=w280, y=u32 30) -> (x+y=w285:u32)
            n127 = dll-call lib="user32.dll" fn="SendMessageA"(error in=w282, "hwnd"=w281, "msg"=w285, "wParam"=w286, "lparam"=w286) -> (error out=w278:errorcluster)  [unwired: 7 in, 1 out]
            n128 = call "WM_CAP - Clipboard to LV.vi"("error in (no error)"=w278, "Erase Clipboard?"=FALSE) -> ("LV_Image"=w276:T7, "error out"=w277:errorcluster)  [unwired: 12 in]
            n129 = call "WM_CAP - Snap Window.vi"("image data"=w276) -> ()  [unwired: 15 in]
            n130 = Bundle By Name(cluster=w283, "Error"=w277) -> (w279:T3)
          }
          event "Frame to BMP": Value Change {
            n131 = event-data() -> ()  [unwired: 1 in, 1 out]
            n132 = call "File Dialog"("prompt"="Save...", "button label"="Save", "pattern (all files)"="*.bmp" ("pattern label"), "pattern label"="Bitmap Files" ("pattern (all files)")) -> ("selected path"=w292:path, "error out"=w291:errorcluster)  [unwired: 8 in, 2 out]
            n133 = case shown="No Error" w291 {
              tunnel: w294 -> [w305 w306]
              tunnel: [w304 w306] -> w293
              tunnel: w292 -> [w295 _]
              frame No Error {
                # "WM_CAP_FILE_SAVEDIBA"
                n134 = Unbundle By Name(w305) -> ("Error"=w299:errorcluster, "hwnd"=w298:u32, "WM_CAP_START"=w297:u32)
                n135 = Add(x=w297, y=u32 25) -> (x+y=w301:u32)
                n136 = Path To String(path=w295) -> (string=w302:string)
                n137 = dll-call lib="user32.dll" fn="SendMessageA"(error in=w299, "hwnd"=w298, "msg"=w301, "wParam"=u32 0 ("msg"), "lparam"=w302) -> (error out=w296:errorcluster)  [unwired: 7 in, 1 out]
                n138 = Bundle By Name(cluster=w305, "Error"=w296) -> (w304:T3)
              }
              frame Error {
              }
            }
          }
          event "Capture": Value Change {
            n139 = event-data() -> ("NewVal"=w307:bool)  [unwired: 1 in]
            n140 = case shown="True" w307 {
              tunnel: w309 -> [w315 w328]
              tunnel: [w311 w324] -> w308
              frame False {
                # "WM_CAP_STOP"
                n141 = Unbundle By Name(w315) -> ("Error"=w314:errorcluster, "hwnd"=w313:u32, "WM_CAP_START"=w312:u32)
                n142 = Add(x=w312, y=u32 68) -> (x+y=w317:u32)
                n143 = dll-call lib="user32.dll" fn="SendMessageA"(error in=w314, "hwnd"=w313, "msg"=w317, "wParam"=u32 0 ("msg"), "lparam"=u32 0 ("msg")) -> (error out=w310:errorcluster)  [unwired: 7 in, 1 out]
                n144 = Bundle By Name(cluster=w315, "Error"=w310) -> (w311:T3)
              }
              frame True {
                w336 = T8 {"dwRequestMicroSecPerFrame"=0, "fMakeUserHitOKToCapture"=0, "wPercentDropForError"=0, "fYield"=0, "dwIndexSize"=0, "wChunkGranularity"=0, "fUsingDOSMemory"=0, "wNumVideoRequested"=0, "fCaptureAudio"=0, "wNumAudioRequested"=0, "vKeyAbort"=0, "fAbortLeftMouse"=0, "fAbortRightMouse"=0, "fLimitEnabled"=0, "wTimeLimit"=0, "fMCIControl"=0, "fStepMCIDevice"=0, "dwMCIStartTime"=0, "dwMCIStopTime"=0, " fStepCaptureAt2x"=0, "wStepCaptureAverageFrames"=0, "dwAudioBufferSize"=0, "fDisableWriteCache"=0, "AVStreamMaster"=0}  # CAPTUREPARMS
                w333 = u32 0 ("msg")
                # "typedef struct {\n  DWORD dwRequestMicroSecPerFrame;\n  BOOL  fMakeUserHitOKToCapture;\n  UINT  wPercentDropForError;\n  BOOL  fYield;\n  DWORD dwIndexSize;\n  UINT  wChunkGranularity;\n  BOOL  fUsingDOSMemory;\n  UINT  wNumVideoRequested;\n  BOOL  fCaptureAudio;\n  UINT  wNumAudioRequested;\n  UINT  vKeyAbort;\n  BOOL  fAbortLeftMouse;\n  BOOL  fAbortRightMouse;\n  BOOL  fLimitEnabled;\n  UINT  wTimeLimit;\n  BOOL  fMCIControl;\n  BOOL  fStepMCIDevice;\n  DWORD dwMCIStartTime;\n  DWORD dwMCIStopTime;\n  BOOL  fStepCaptureAt2x;\n  UINT  wStepCaptureAverageFrames;\n  DWORD dwAudioBufferSize;\n  BOOL  fDisableWriteCache;\n  UINT  AVStreamMaster;\n} CAPTUREPARMS;"
                # "WM_CAP_GET_SEQUENCE_SETUP"
                # "WM_CAP_SEQUENCE"
                n145 = Unbundle By Name(w328) -> ("Error"=w327:errorcluster, "hwnd"=w326:u32, "WM_CAP_START"=w325:u32, "Capture FPS"=w323:dbl)
                n146 = Reciprocal(x=w323) -> (1/x=w351:dbl)
                n147 = Multiply(x=w351, y=1000000.0) -> (x*y=w353:dbl)
                n148 = Flatten To String(anything=w336, prepend array or string size? (T)=FALSE) -> (data string=w334:string)  [unwired: 2 in, 2 out]
                n149 = To Unsigned Long Integer(number=w353) -> (unsigned 32bit integer=w354:u32)
                n150 = Add(x=w325, y=u16 65) -> (x+y=w330:u32)
                n151 = String Length(string=w334) -> (length=w343:i32)
                n152 = dll-call lib="user32.dll" fn="SendMessageA"(error in=w327, "hwnd"=w326, "msg"=w330, "wParam"=w343, w336) -> (error out=w337:errorcluster, "hwnd"=w339:u32, w344:T8)  [unwired: 5 in, 1 out]
                n153 = Bundle By Name(cluster=w344, "dwRequestMicroSecPerFrame"=w354, "fYield"=u32 1, "dwIndexSize"=u32 324000, "fAbortLeftMouse"=u32 0, "fAbortRightMouse"=u32 0, "fLimitEnabled"=u32 0) -> (w345:T8)
                n154 = Add(x=w325, y=u16 64) -> (x+y=w342:u32)
                n155 = dll-call lib="user32.dll" fn="SendMessageA"(error in=w337, "hwnd"=w339, "msg"=w342, "wParam"=w343, w345) -> (error out=w338:errorcluster, "hwnd"=w340:u32)  [unwired: 6 in, 1 out]
                n156 = Add(x=w325, y=u16 62) -> (x+y=w332:u32)
                n157 = dll-call lib="user32.dll" fn="SendMessageA"(error in=w338, "hwnd"=w340, "msg"=w332, "wParam"=w333, "lparam"=w333) -> (error out=w322:errorcluster)  [unwired: 7 in, 1 out]
                n158 = call "WM_CAP - Get Camera Name.vi"("error in (no error)"=w322) -> ("FriendlyName"=w320:string, "error out"=w321:errorcluster)  [unwired: 12 in, 1 out]
                n159 = Bundle By Name(cluster=w328, "Camera"=w320, "Error"=w321) -> (w324:T3)
              }
            }
          }
          event "Export": Value Change {
            n160 = event-data() -> ()  [unwired: 1 in, 1 out]
            n161 = call "File Dialog2"("prompt"="Export...", "button label"="Export", "pattern (all files)"="*.avi" ("pattern label"), "pattern label"="Video Files" ("pattern (all files)")) -> ("selected path"=w358:path, "error out"=w357:errorcluster)  [unwired: 8 in, 2 out]
            n162 = case shown="No Error" w357 {
              tunnel: w362 -> [w369 w376]
              tunnel: [w365 w376] -> w361
              tunnel: w358 -> [w363 _]
              frame No Error {
                # "WM_CAP_FILE_SAVEAS"
                n163 = Unbundle By Name(w369) -> ("Error"=w368:errorcluster, "hwnd"=w367:u32, "WM_CAP_START"=w366:u32)
                n164 = call <vilib>:"Set Busy.vi"("error in (no error)"=w368) -> ("error out"=w374:errorcluster)  [unwired: 9 in, 1 out]
                n165 = Add(x=w366, y=u32 23) -> (x+y=w371:u32)
                n166 = Path To String(path=w363) -> (string=w373:string)
                n167 = dll-call lib="user32.dll" fn="SendMessageA"(error in=w374, "hwnd"=w367, "msg"=w371, "wParam"=u32 0 ("msg"), "lparam"=w373) -> (error out=w375:errorcluster)  [unwired: 7 in, 1 out]
                n168 = call <vilib>:"Unset Busy.vi"("error in (no error)"=w375) -> ("error out"=w364:errorcluster)  [unwired: 10 in]
                n169 = Bundle By Name(cluster=w369, "Error"=w364) -> (w365:T3)
              }
              frame Error {
              }
            }
          }
          event "Preview": Value Change {
            # "WM_CAP_SET_PREVIEWRATE"
            # "WM_CAP_SET_PREVIEW"
            n170 = event-data() -> ()  [unwired: 1 in, 1 out]
            n171 = Unbundle By Name(w382) -> ("Preview FPS"=w386:dbl, "CAPSTATUS.fLiveWindow"=w384:u32, "Error"=w388:errorcluster, "hwnd"=w387:u32, "WM_CAP_START"=w385:u32)
            n172 = Not Equal To 0?(x=w384) -> (x != 0?=w380:bool)
            n173 = Add(x=w385, y=u32 52) -> (x+y=w393:u32)
            n174 = case shown="False" w380 {
              tunnel: w393 -> [w406 _]
              tunnel: [w401 w409] -> w394
              tunnel: w388 -> [w400 w409]
              tunnel: w387 -> [w399 w408]
              tunnel: [w398 w408] -> w395
              tunnel: w386 -> [w397 _]
              tunnel: [u32 1 ("wParam") _] -> w383
              frame False {
                n175 = Reciprocal(x=w397) -> (1/x=w405:dbl)
                n176 = Multiply(x=w405, y=1000.0) -> (x*y=w403:dbl)
                n177 = To Unsigned Long Integer(number=w403) -> (unsigned 32bit integer=w402:u32)
                n178 = dll-call lib="user32.dll" fn="SendMessageA"(error in=w400, "hwnd"=w399, "msg"=w406, "wParam"=w402, "lparam"=u32 0) -> (error out=w401:errorcluster, "hwnd"=w398:u32)  [unwired: 6 in, 1 out]
              }
              frame True {
              }
            }
            n179 = Add(x=w385, y=u32 50) -> (x+y=w390:u32)
            n180 = dll-call lib="user32.dll" fn="SendMessageA"(error in=w394, "hwnd"=w395, "msg"=w390, "wParam"=w383, "lparam"=u32 0) -> (error out=w379:errorcluster)  [unwired: 7 in, 1 out]
            n181 = call "WM_CAP - Get Camera Name.vi"("error in (no error)"=w379) -> ("FriendlyName"=w377:string, "error out"=w378:errorcluster)  [unwired: 12 in, 1 out]
            n182 = Bundle By Name(cluster=w382, "Camera"=w377, "Error"=w378) -> (w381:T3)
          }
          event "Fit Window": Value Change {
            # "WM_CAP_SET_SCALE"
            n183 = event-data() -> ()  [unwired: 1 in, 1 out]
            n184 = Unbundle By Name(w415) -> ("CAPSTATUS.fScale"=w411:u32, "Error"=w414:errorcluster, "hwnd"=w413:u32, "WM_CAP_START"=w412:u32)
            n185 = Not Equal To 0?(x=w411) -> (x != 0?=w410:bool)
            n186 = Select(t=u32 0 ("wParam"), s=w410, f=u32 1 ("wParam")) -> (s? t:f=w420:u32)
            n187 = Add(x=w412, y=u16 53) -> (x+y=w417:u32)
            n188 = dll-call lib="user32.dll" fn="SendMessageA"(error in=w414, "hwnd"=w413, "msg"=w417, "wParam"=w420, "lparam"=u32 0) -> ()  [unwired: 7 in, 2 out]
          }
        }
      }
    }
  }
